vi "Triangle global info.vi"() -> ()   [LabVIEW 2012]
panel:
  in  "Triangle Info":T1
  # "Operator Info"
  # "R"
  # "L"
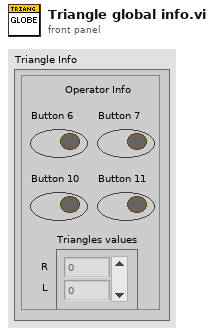
[diagram p1: front panel]
types:
  T1 = cluster{"Button 6":bool, "Button 7":bool, "Button 10":bool, "Button 11":bool, "Triangles values":dbl[]}
diagram:
